vi "INIT.vi"(8 "error in (no error)":errorcluster, 11 "DelayLineLS4 in":refnum<class "DLLS4.lvclass">) -> (0 "error out":errorcluster, 3 "DelayLineLS4 out":refnum<class "DLLS4.lvclass">)   [LabVIEW 2018, in "DLLS4.lvclass"]
uses:
  DLLS4.lvclass
  C:/Users/Sergey Denisov/Documents/REPS/TRANCON/Classes/GeneralFunctionality/GeneralFunctionality.lvclass
  GeneralFunctionality/GeneralFunctionality.lvclass/GeneralFunctionality.ctl
  dependecies/ControlsVIs/Clusters-def/SERVER-Commands.ctl
  dependecies/ControlsVIs/Clusters-def/Message types.ctl
  Message/Message.lvclass
  Control/Control-Server/Control-Server.lvclass
  GeneralFunctionality/GeneralFunctionality.lvclass
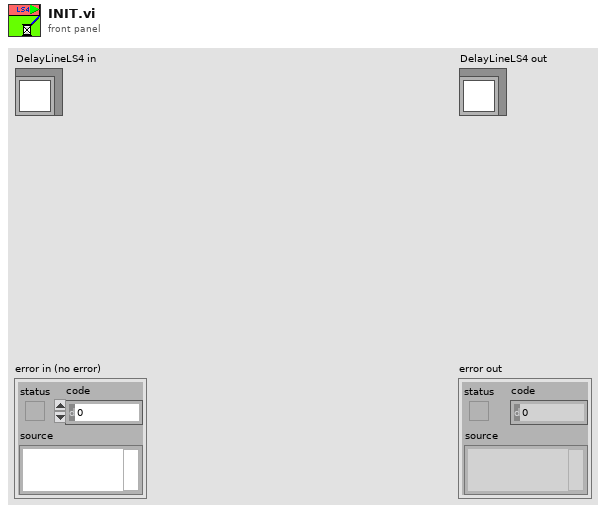
[diagram p1: front panel]
types:
  T1 = typedef "Message types.ctl" = string
  T2 = typedef "Control-Server.lvclass/SERVER-Commands.ctl" = string
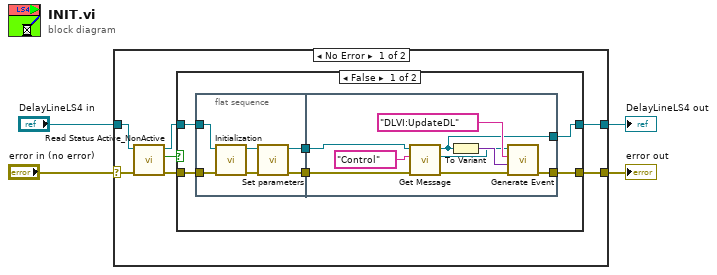
[diagram p0: block diagram]
diagram:
  n1 = case shown="No Error" "error in (no error)" {
    selector: "error in (no error)" -> [w8 w35]
    tunnel: "DelayLineLS4 in" -> [w9 w36]
    tunnel: [w11 w36] -> w2
    tunnel: [w10 w35] -> w1
    frame No Error {
      n2 = call "Read Status Active_NonActive.vi"("error in (no error)"=w8, "GeneralFunctionality in"=w9) -> ("error out"=w5:errorcluster, "Status Active/NonActive"=w7:bool, "GeneralFunctionality out"=w6:refnum<class "DLLS4.lvclass">)  [unwired: 7 in]
      n3 = case shown="False" w7 {
        tunnel: [w12 w34] -> w11
        tunnel: [w15 w33] -> w10
        tunnel: w6 -> [w17 w34]
        tunnel: w5 -> [w16 w33]
        frame False {
          n4 = flat-sequence {
            tunnel: w17 -> [w21]
            tunnel: w16 -> [w20]
            tunnel: [w19] -> w14
            tunnel: [w18] -> w13
            tunnel: w14 -> [w30]
            tunnel: w13 -> [w26]
            tunnel: [w28] -> w15
            tunnel: [w25] -> w12
            frame #0 {
              n5 = call-dynamic "Initialization.vi"("error in (no error)"=w20, "DelayLineLS4 in"=w21) -> ("error out"=w23:errorcluster, "DelayLineLS4 out"=w22:refnum<class "DLLS4.lvclass">)  [unwired: 8 in]
              n6 = call-dynamic "Set parameters.vi"("error in (no error)"=w23, "DelayLineLS4 en entrée"=w22) -> ("error out"=w19:errorcluster, "DelayLineLS4 en sortie"=w18:refnum<class "DLLS4.lvclass">)  [unwired: 8 in]
            }
            frame #1 {
              n7 = call "Get Message.vi"("error in (no error)"=w30, "Message type"=T1 "Control", "GeneralFunctionality en entrée"=w26) -> ("error out"=w29:errorcluster, "Message.lvclass"=w27:refnum<class "Message.lvclass">, "GeneralFunctionality en sortie"=w25:refnum<class "DLLS4.lvclass">)  [unwired: 6 in]
              n8 = To Variant(anything=w25) -> (Variant=w32:variant)
              n9 = call "Generate Event.vi"("error in (no error)"=w29, "Data"=w32, "Command"=T2 "DLVI:UpdateDL", "Message en entrée"=w27) -> ("error out"=w28:errorcluster)  [unwired: 6 in, 1 out]
            }
          }
        }
        frame True {
        }
      }
    }
    frame Error {
    }
  }
  "error out" <- w1
  "DelayLineLS4 out" <- w2
